vi "ActOnEnable.vi"(0 "ActionLvDialog in":refnum<class "ActionLvDialog.lvclass">, 1 "Data":variant, 5 "error in (no error)":errorcluster) -> (14 "ActionLvDialog out":refnum<class "ActionLvDialog.lvclass">, 19 "error out":errorcluster)   [LabVIEW 2017, in "ActionLvDialog.lvclass"]
doc: "Base class implementation (empty)."
uses:
  ActionLvDialog.lvclass
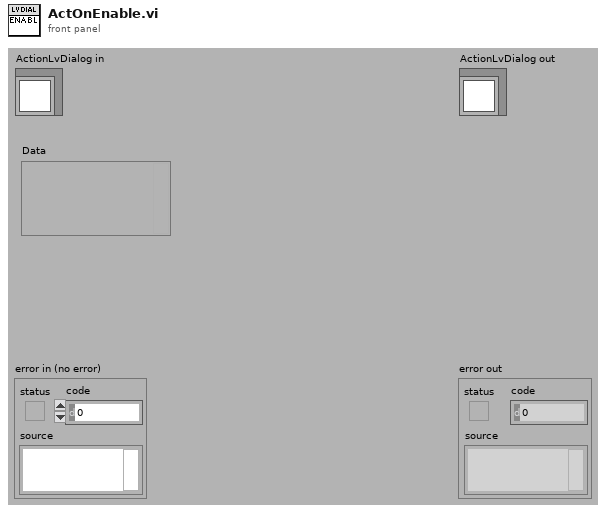
[diagram p1: front panel]
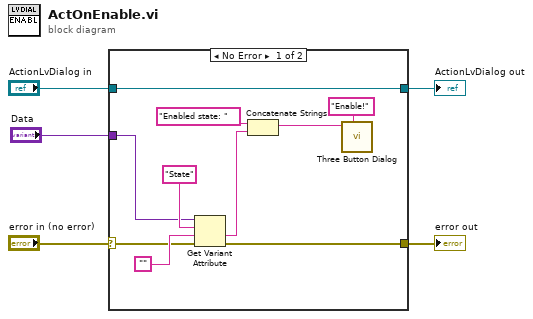
[diagram p0: block diagram]
diagram:
  n1 = case shown="No Error" "error in (no error)" {
    selector: "error in (no error)" -> [w13 w16]
    tunnel: "ActionLvDialog in" -> [w6 w17]
    tunnel: "Data" -> [w12 _]
    tunnel: [w10 w16] -> w2
    tunnel: [w6 w17] -> w1
    frame No Error {
      n2 = Get Variant Attribute(Variant=w12, name="State", default value (empty Variant)="", error in=w13) -> (value=w8:string, error out=w10:errorcluster)  [unwired: 2 out]
      n3 = Concatenate Strings("Enabled state: " ("string"), w8) -> (w7:string)
      n4 = call <vilib>:"Three Button Dialog.vi"("Window Title (\"\")"="Enable!" ("Window Title (\"\")"), "message"=w7) -> ()  [unwired: 9 in, 1 out]
    }
    frame Error {
    }
  }
  "error out" <- w2
  "ActionLvDialog out" <- w1
